vi "AddSlowAO.vi"(1 "RT Actions (without slowAO)":T4=[{"Macro Instructions"=[{"Duration (s)"=0.1, "Steps"=1, "Changes"=[TRUE, FALSE], "Triggers"=[FALSE, FALSE, FALSE, FALSE, FALSE, FALSE, FALSE, FALSE, FALSE, FALSE, FALSE, FALSE, FALSE, FALSE, FALSE, FALSE, FALSE, FALSE, FALSE, FALSE, FALSE, FALSE, FALSE, FALSE, FALSE, FALSE, FALSE, FALSE, FALSE, FALSE, FALSE, FALSE, FALSE, FALSE, FALSE, FALSE, FALSE, FALSE], "RAW cmds 2D"=[[0, 0, 0, 0, 0, 0, 0, 0], [0, 0, 0, 0, 0, 0, 0, 0]]}], "Slow AO Array"=[], "Duration (s)"=0.1, "Toggle"=TRUE}, {"Macro Instructions"=[{"Duration (s)"=0.1, "Steps"=1, "Changes"=[TRUE, FALSE], "Triggers"=[FALSE, FALSE, FALSE, FALSE, FALSE, FALSE, FALSE, FALSE, FALSE, FALSE, FALSE, FALSE, FALSE, FALSE, FALSE, FALSE, FALSE, FALSE, FALSE, FALSE, FALSE, FALSE, FALSE, FALSE, FALSE, FALSE, FALSE, FALSE, FALSE, FALSE, FALSE, FALSE, FALSE, FALSE, FALSE, FALSE, FALSE, FALSE], "RAW cmds 2D"=[[0, 0, 0, 0, 0, 0, 0, 0], [0, 0, 0, 0, 0, 0, 0, 0]]}], "Slow AO Array"=[], "Duration (s)"=0.1, "Toggle"=TRUE}, {"Macro Instructions"=[{"Duration (s)"=0.1, "Steps"=1, "Changes"=[TRUE, FALSE], "Triggers"=[FALSE, FALSE, FALSE, FALSE, FALSE, FALSE, FALSE, FALSE, FALSE, FALSE, FALSE, FALSE, FALSE, FALSE, FALSE, FALSE, FALSE, FALSE, FALSE, FALSE, FALSE, FALSE, FALSE, FALSE, FALSE, FALSE, FALSE, FALSE, FALSE, FALSE, FALSE, FALSE, FALSE, FALSE, FALSE, FALSE, FALSE, FALSE], "RAW cmds 2D"=[[0, 0, 0, 0, 0, 0, 0, 0], [0, 0, 0, 0, 0, 0, 0, 0]]}], "Slow AO Array"=[], "Duration (s)"=0.1, "Toggle"=TRUE}] {"Slow AO Array"."Duration, Gain, NewVal" format="%#_3g"}, 2 "DAC cmds":string[](array[string])=["Action 0\n.05\tao5\t15\t-130\t130\t5.000000E+1\r\n.05\tao6\t200\t0\t950\t0.000000E+0\r\n.05\tao7\t500\t0\t3500\t0.000000E+0\r\n", "Action 1\n0.1\tinbit\t-1\t0\t7\t1.000000E+0\r\n", "Action 2\n.05\tao5\t15\t-130\t130\t0.000000E+0\r\n.05\tao6\t200\t0\t950\t0.000000E+0\r\n.05\tao7\t500\t0\t3500\t0.000000E+0\r\n"]) -> (0 "RT Actions":T1[](array[typedef])=[{"Macro Instructions"=[{"Duration (s)"=0.1, "Steps"=1, "Changes"=[TRUE, FALSE], "Triggers"=[FALSE, FALSE, FALSE, FALSE, FALSE, FALSE, FALSE, FALSE, FALSE, FALSE, FALSE, FALSE, FALSE, FALSE, FALSE, FALSE, FALSE, FALSE, FALSE, FALSE, FALSE, FALSE, FALSE, FALSE, FALSE, FALSE, FALSE, FALSE, FALSE, FALSE, FALSE, FALSE, FALSE, FALSE, FALSE, FALSE, FALSE, FALSE], "RAW cmds 2D"=[[0, 0, 0, 0, 0, 0, 0, 0], [0, 0, 0, 0, 0, 0, 0, 0]]}], "Slow AO Array"=[{"ao line"="ao5", "Duration, Gain, NewVal"=[0.05, 15.0, -130.0, 130.0, 50.0]}, {"ao line"="ao6", "Duration, Gain, NewVal"=[0.05, 200.0, 0.0, 950.0, 0.0]}, {"ao line"="ao7", "Duration, Gain, NewVal"=[0.05, 500.0, 0.0, 3500.0, 0.0]}], "Duration (s)"=0.1, "Toggle"=TRUE}, {"Macro Instructions"=[{"Duration (s)"=0.1, "Steps"=1, "Changes"=[TRUE, FALSE], "Triggers"=[FALSE, FALSE, FALSE, FALSE, FALSE, FALSE, FALSE, FALSE, FALSE, FALSE, FALSE, FALSE, FALSE, FALSE, FALSE, FALSE, FALSE, FALSE, FALSE, FALSE, FALSE, FALSE, FALSE, FALSE, FALSE, FALSE, FALSE, FALSE, FALSE, FALSE, FALSE, FALSE, FALSE, FALSE, FALSE, FALSE, FALSE, FALSE], "RAW cmds 2D"=[[0, 0, 0, 0, 0, 0, 0, 0], [0, 0, 0, 0, 0, 0, 0, 0]]}], "Slow AO Array"=[{"ao line"="inbit", "Duration, Gain, NewVal"=[0.1, -1.0, 0.0, 7.0, 1.0]}], "Duration (s)"=0.1, "Toggle"=TRUE}, {"Macro Instructions"=[{"Duration (s)"=0.1, "Steps"=1, "Changes"=[TRUE, FALSE], "Triggers"=[FALSE, FALSE, FALSE, FALSE, FALSE, FALSE, FALSE, FALSE, FALSE, FALSE, FALSE, FALSE, FALSE, FALSE, FALSE, FALSE, FALSE, FALSE, FALSE, FALSE, FALSE, FALSE, FALSE, FALSE, FALSE, FALSE, FALSE, FALSE, FALSE, FALSE, FALSE, FALSE, FALSE, FALSE, FALSE, FALSE, FALSE, FALSE], "RAW cmds 2D"=[[0, 0, 0, 0, 0, 0, 0, 0], [0, 0, 0, 0, 0, 0, 0, 0]]}], "Slow AO Array"=[{"ao line"="ao5", "Duration, Gain, NewVal"=[0.05, 15.0, -130.0, 130.0, 0.0]}, {"ao line"="ao6", "Duration, Gain, NewVal"=[0.05, 200.0, 0.0, 950.0, 0.0]}, {"ao line"="ao7", "Duration, Gain, NewVal"=[0.05, 500.0, 0.0, 3500.0, 0.0]}], "Duration (s)"=0.1, "Toggle"=TRUE}] {"Slow AO Array"."Duration, Gain, NewVal" format="%#_3g"})   [LabVIEW 2018]
uses:
  RT Actions.ctl
  RT/ActionCluster.ctl
  RT/Instructions_RT.ctl
  RT/ParameterSubCluster.ctl
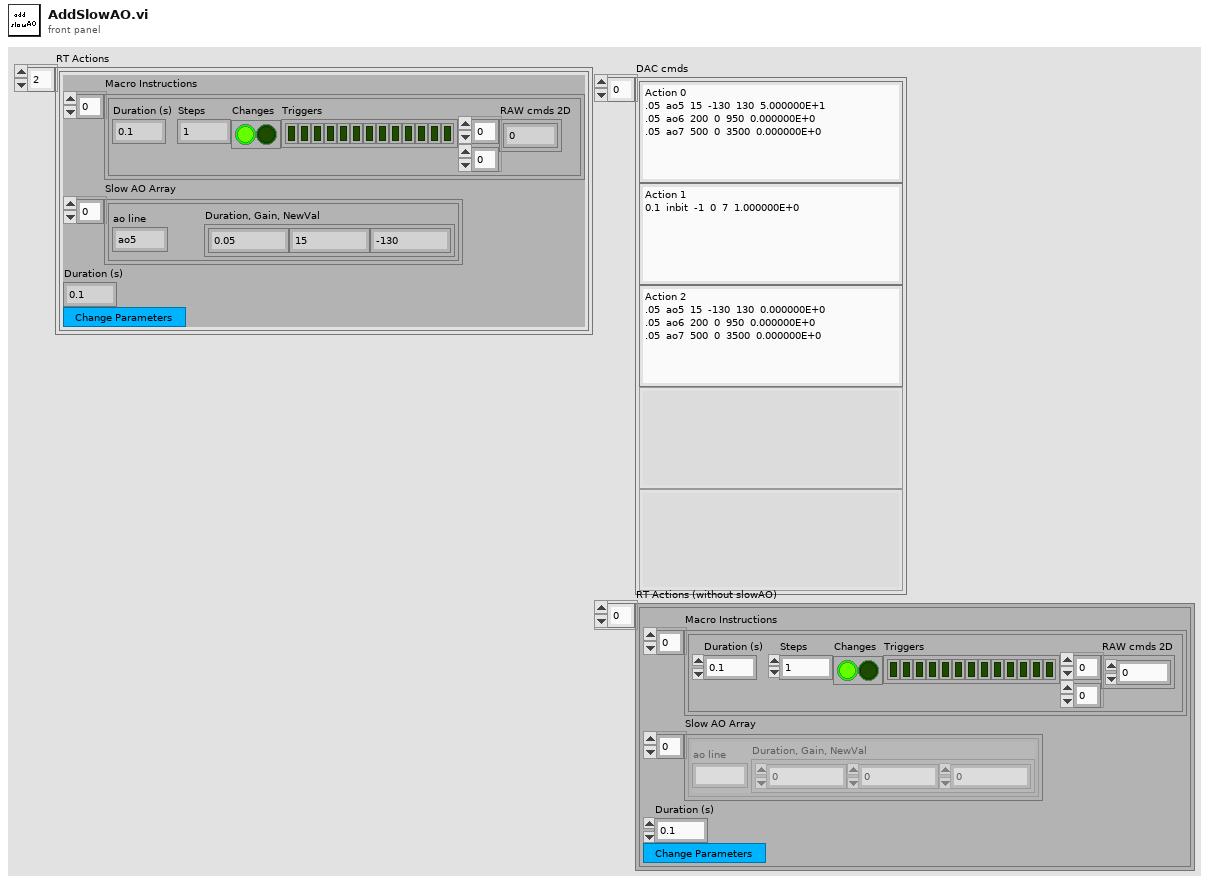
[diagram p1: front panel]
types:
  T1 = typedef "ActionCluster.ctl" = cluster{"Macro Instructions":T2, "Slow AO Array":T3, "Duration (s)":dbl, "Toggle":bool}
  T2 = typedef "Instructions_RT.ctl" = cluster{"Duration (s)":dbl, "Steps":i32, "Changes":bool[], "Triggers":bool[], "RAW cmds 2D":i16[][]}[]
  T3 = typedef "ParameterSubCluster.ctl" = cluster{"ao line":string, "Duration, Gain, NewVal":dbl[]}[]
  T4 = typedef "RT Actions.ctl" = T1[]
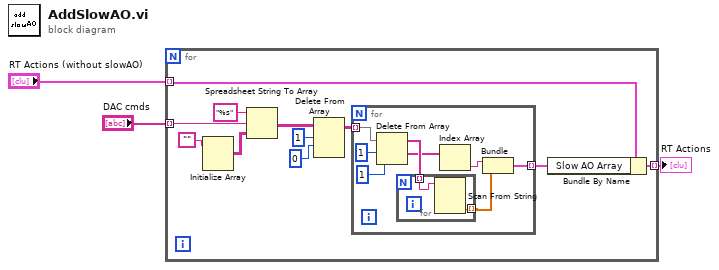
[diagram p0: block diagram]
diagram:
  n1 = for {
    tunnel: "RT Actions (without slowAO)" -> [w4] mode=indexing
    tunnel: "DAC cmds" -> [w14] mode=indexing
    tunnel: [w6] -> w1 mode=indexing
    n2 = Initialize Array("") -> (w11:string[][])  [unwired: 2 in]
    n3 = Spreadsheet String To Array(format string="%s", spreadsheet string=w14, array type (2D Dbl)=w11) -> (array=w10:string[][])  [unwired: 1 in]
    n4 = Delete From Array(array=w10, length=1, index (row)=0) -> (array with subset deleted=w8:string[][])  [unwired: 1 in, 1 out]
    n5 = for {
      tunnel: w8 -> [w22] mode=indexing
      tunnel: [w15] -> w7 mode=indexing
      n6 = Delete From Array(array=w22, length=1, index=1) -> (deleted portion=w17:string[], array with subset deleted=w19:string[])
      n7 = for {
        tunnel: w19 -> [w24] mode=indexing
        tunnel: [w23] -> w18 mode=indexing
        n8 = Scan From String(input string=w24) -> (output 1=w23:dbl)  [unwired: 4 in, 3 out]
      }
      n9 = Index Array(array=w17) -> (element=w16:string)  [unwired: 1 in]
      n10 = Bundle(w16, w18) -> (w15:cluster{string, dbl[]})  [unwired: 1 in]
    }
    n11 = Bundle By Name(cluster=w4, "Slow AO Array"=w7) -> (w6:T1)
  }
  "RT Actions" <- w1
